vi "GRNF_ColorSensor.vi"(7 "RefNum Name":string="My Motor RefNum") -> (0 "Error":errorcluster, 3 "Device Reference":T1={"I2CDevRef"={"DevStatus"={"status"=FALSE, "code"=0, "source"=""}, "Device Address"=0, "Handle"=0, "I2C Bus"=enum."Invalid"}} {"I2CDevRef"."Device Address" format="%.0x"})   [LabVIEW 2020]
doc: "This VI loads a REV Color Sensor v3 refnum on code boot and then stores it in memory so that the information does not have to be queried on subsequent loop cycles. This VI is configured for polymorphic use."
uses:
  <vilib>/Rock Robotics/SystemInterfaces/i2clib/i2c_bus.ctl
  <vilib>/Rock Robotics/WPI/I2C/WPI_I2CDevRef.ctl
  <vilib>/Rock Robotics/WPI/ThirdParty/REV Robotics/REVLib/Typedef/Color Sensor V3 DevRef.ctl
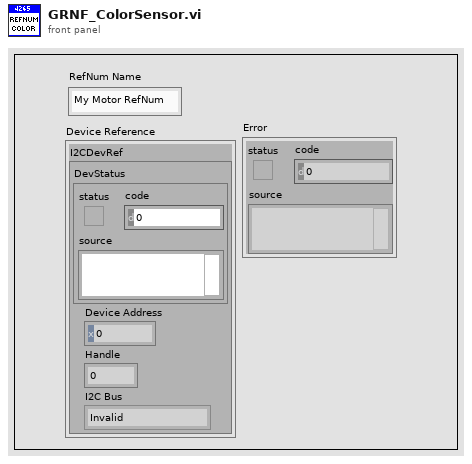
[diagram p1: front panel]
types:
  T1 = typedef "Color Sensor V3 DevRef.ctl" = cluster{"I2CDevRef":T2}
  T2 = typedef "WPI_I2CDevRef.ctl" = cluster{"DevStatus":errorcluster, "Device Address":u8, "Handle":i32, "I2C Bus":T3}
  T3 = typedef "i2c_bus.ctl" = enum16{"I2C On-Board", "I2C MXP", "Invalid"}
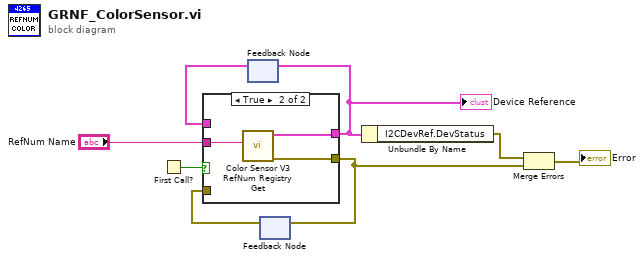
[diagram p0: block diagram]
diagram:
  n1 = First Call?() -> (First Call?: T/F=w8:bool)
  n2 = feedback #1() -> (w7:T1)  [unwired: 1 in]
  n3 = feedback #2() -> (w5:errorcluster)  [unwired: 1 in]
  n4 = case shown="True" w8 {
    tunnel: [w10 w13] -> w3
    tunnel: w7 -> [w10 _]
    tunnel: "RefNum Name" -> [_ w11]
    tunnel: [w9 w12] -> w2
    tunnel: w5 -> [w9 _]
    frame False {
    }
    frame True {
      n5 = call <vilib>:"Color Sensor V3 RefNum Registry Get.vi"("refnum name"=w11) -> ("error out"=w12:errorcluster, "ColorSensorDevRef"=w13:T1)  [unwired: 9 in]
    }
  }
  "Device Reference" <- w3
  n6 = feedback-in #1(w3) -> ()
  n7 = feedback-in #2(w2) -> ()
  n8 = Unbundle By Name(w3) -> ("I2CDevRef.DevStatus"=w4:errorcluster)
  n9 = Merge Errors(w4, w2) -> (→"Error":errorcluster)
